vi "flinger_getInputs.vi"() -> ()   [LabVIEW 2013]
uses:
  util/joystick_vals.ctl
  <vilib>/Rock Robotics/WPI/Joystick/WPI_JoystickButtonState.ctl
  flinger_inputs.ctl
panel:
  in  "Flinger Inputs 2":T1
  out "Flinger Inputs":T1
  in  "Joysticks":T2
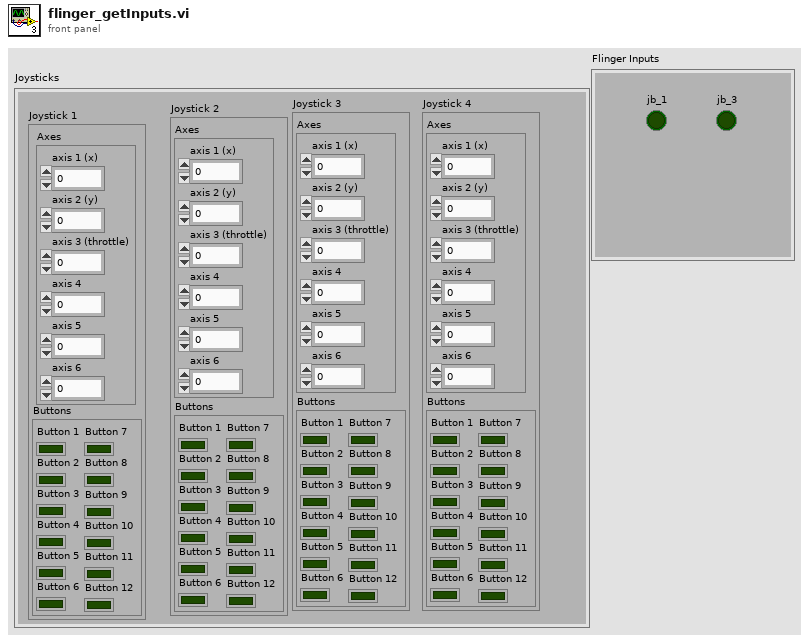
[diagram p1: front panel]
types:
  T1 = typedef "flinger_inputs.ctl" = cluster{"jb_1":bool, "jb_3":bool}
  T2 = typedef "joystick_vals.ctl" = cluster{"Joystick 1":cluster{"Axes":cluster{"axis 1 (x)":dbl, "axis 2 (y)":dbl, "axis 3 (throttle)":dbl, "axis 4":dbl, "axis 5":dbl, "axis 6":dbl}, "Buttons":T3}, "Joystick 2":cluster{"Axes":cluster{"axis 1 (x)":dbl, "axis 2 (y)":dbl, "axis 3 (throttle)":dbl, "axis 4":dbl, "axis 5":dbl, "axis 6":dbl}, "Buttons":T3}, "Joystick 3":cluster{"Axes":cluster{"axis 1 (x)":dbl, "axis 2 (y)":dbl, "axis 3 (throttle)":dbl, "axis 4":dbl, "axis 5":dbl, "axis 6":dbl}, "Buttons":T3}, "Joystick 4":cluster{"Axes":cluster{"axis 1 (x)":dbl, "axis 2 (y)":dbl, "axis 3 (throttle)":dbl, "axis 4":dbl, "axis 5":dbl, "axis 6":dbl}, "Buttons":T3}}
  T3 = typedef "WPI_JoystickButtonState.ctl" = cluster{"Button 1":bool, "Button 2":bool, "Button 3":bool, "Button 4":bool, "Button 5":bool, "Button 6":bool, "Button 7":bool, "Button 8":bool, "Button 9":bool, "Button 10":bool, "Button 11":bool, "Button 12":bool}
  T4 = cluster{"Axes":cluster{"axis 1 (x)":dbl, "axis 2 (y)":dbl, "axis 3 (throttle)":dbl, "axis 4":dbl, "axis 5":dbl, "axis 6":dbl}, "Buttons":T3}
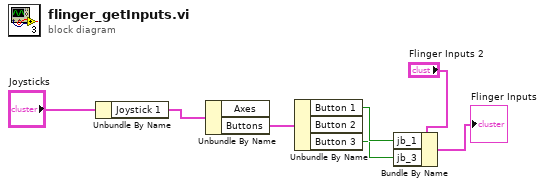
[diagram p0: block diagram]
diagram:
  n1 = Unbundle By Name("Joysticks") -> ("Joystick 1"=w6:T4)
  n2 = Unbundle By Name(w6) -> ("Buttons"=w5:T3)  [unwired: 1 out]
  n3 = Unbundle By Name(w5) -> ("Button 1"=w2:bool, "Button 3"=w1:bool)  [unwired: 1 out]
  n4 = Bundle By Name(cluster="Flinger Inputs 2", "jb_1"=w2, "jb_3"=w1) -> (→"Flinger Inputs":T1)
